vi "App - analyze RUS V6.vi"() -> ()   [LabVIEW 2018] (continued)
ember_2014\\091714\\45.19600K_500_2500_2.10000V_0.00000T_Sep17-2014__13-27-32_001_091714.bin", "mod time(min)"=58230327.53333333, "file format"=enum."binary", "power(V)"=2.1, "Magn Field(T) "=0.0}, {"temperature"=45.12, "temperature str"="45.12000", "file path"=path "D:/Data/Ultrasound/LSCO/LSCO22__130814c/5_Cooling_2nd_try/September_2014/091714/45.12000K_500_2500_2.10000V_0.00000T_Sep17-2014__13-28-51_001_091714.bin", "last mod"=timestamp(3493819731 s since 1904-01-01), "file name str"="D:\\Data\\Ultrasound\\LSCO\\LSCO22__130814c\\5_Cooling_2nd_try\\September_2014\\091714\\45.12000K_500_2500_2.10000V_0.00000T_Sep17-2014__13-28-51_001_091714.bin", "mod time(min)"=58230328.85, "file format"=enum."binary", "power(V)"=2.1, "Magn Field(T) "=0.0}, {"temperature"=45.046, "temperature str"="45.04600", "file path"=path "D:/Data/Ultrasound/LSCO/LSCO22__130814c/5_Cooling_2nd_try/September_2014/091714/45.04600K_500_2500_2.10000V_0.00000T_Sep17-2014__13-30-10_001_091714.bin", "last mod"=timestamp(3493819810 s since 1904-01-01), "file name str"="D:\\Data\\Ultrasound\\LSCO\\LSCO22__130814c\\5_Cooling_2nd_try\\September_2014\\091714\\45.04600K_500_2500_2.10000V_0.00000T_Sep17-2014__13-30-10_001_091714.bin", "mod time(min)"=58230330.166666664, "file format"=enum."binary", "power(V)"=2.1, "Magn Field(T) "=0.0}, {"temperature"=44.972, "temperature str"="44.97200", "file path"=path "D:/Data/Ultrasound/LSCO/LSCO22__130814c/5_Cooling_2nd_try/September_2014/091714/44.97200K_500_2500_2.10000V_0.00000T_Sep17-2014__13-31-30_001_091714.bin", "last mod"=timestamp(3493819890 s since 1904-01-01), "file name str"="D:\\Data\\Ultrasound\\LSCO\\LSCO22__130814c\\5_Cooling_2nd_try\\September_2014\\091714\\44.97200K_500_2500_2.10000V_0.00000T_Sep17-2014__13-31-30_001_091714.bin", "mod time(min)"=58230331.5, "file format"=enum."binary", "power(V)"=2.1, "Magn Field(T) "=0.0}, {"temperature"=44.9, "temperature str"="44.90000", "file path"=path "D:/Data/Ultrasound/LSCO/LSCO22__130814c/5_Cooling_2nd_try/September_2014/091714/44.90000K_500_2500_2.10000V_0.00000T_Sep17-2014__13-32-49_001_091714.bin", "last mod"=timestamp(3493819969 s since 1904-01-01), "file name str"="D:\\Data\\Ultrasound\\LSCO\\LSCO22__130814c\\5_Cooling_2nd_try\\September_2014\\091714\\44.90000K_500_2500_2.10000V_0.00000T_Sep17-2014__13-32-49_001_091714.bin", "mod time(min)"=58230332.81666667, "file format"=enum."binary", "power(V)"=2.1, "Magn Field(T) "=0.0}, {"temperature"=44.826, "temperature str"="44.82600", "file path"=path "D:/Data/Ultrasound/LSCO/LSCO22__130814c/5_Cooling_2nd_try/September_2014/091714/44.82600K_500_2500_2.10000V_0.00000T_Sep17-2014__13-34-09_001_091714.bin", "last mod"=timestamp(3493820049 s since 1904-01-01), "file name str"="D:\\Data\\Ultrasound\\LSCO\\LSCO22__130814c\\5_Cooling_2nd_try\\September_2014\\091714\\44.82600K_500_2500_2.10000V_0.00000T_Sep17-2014__13-34-09_001_091714.bin", "mod time(min)"=58230334.15, "file format"=enum."binary", "power(V)"=2.1, "Magn Field(T) "=0.0}, {"temperature"=44.75, "temperature str"="44.75000", "file path"=path "D:/Data/Ultrasound/LSCO/LSCO22__130814c/5_Cooling_2nd_try/September_2014/091714/44.75000K_500_2500_2.10000V_0.00000T_Sep17-2014__13-35-28_001_091714.bin", "last mod"=timestamp(3493820128 s since 1904-01-01), "file name str"="D:\\Data\\Ultrasound\\LSCO\\LSCO22__130814c\\5_Cooling_2nd_try\\September_2014\\091714\\44.75000K_500_2500_2.10000V_0.00000T_Sep17-2014__13-35-28_001_091714.bin", "mod time(min)"=58230335.46666667, "file format"=enum."binary", "power(V)"=2.1, "Magn Field(T) "=0.0}, {"temperature"=44.678, "temperature str"="44.67800", "file path"=path "D:/Data/Ultrasound/LSCO/LSCO22__130814c/5_Cooling_2nd_try/September_2014/091714/44.67800K_500_2500_2.10000V_0.00000T_Sep17-2014__13-36-47_001_091714.bin", "last mod"=timestamp(3493820207 s since 1904-01-01), "file name str"="D:\\Data\\Ultrasound\\LSCO\\LSCO22__130814c\\5_Cooling_2nd_try\\September_2014\\091714\\44.67800K_500_2500_2.10000V_0.00000T_Sep17-2014__13-36-47_001_091714.bin", "mod time(min)"=58230336.78333333, "file format"=enum."binary", "power(V)"=2.1, "Magn Field(T) "=0.0}, {"temperature"=44.607, "temperature str"="44.60700", "file path"=path "D:/Data/Ultrasound/LSCO/LSCO22__130814c/5_Cooling_2nd_try/September_2014/091714/44.60700K_500_2500_2.10000V_0.00000T_Sep17-2014__13-38-07_001_091714.bin", "last mod"=timestamp(3493820287 s since 1904-01-01), "file name str"="D:\\Data\\Ultrasound\\LSCO\\LSCO22__130814c\\5_Cooling_2nd_try\\September_2014\\091714\\44.60700K_500_2500_2.10000V_0.00000T_Sep17-2014__13-38-07_001_091714.bin", "mod time(min)"=58230338.11666667, "file format"=enum."binary", "power(V)"=2.1, "Magn Field(T) "=0.0}, {"temperature"=44.533, "temperature str"="44.53300", "file path"=path "D:/Data/Ultrasound/LSCO/LSCO22__130814c/5_Cooling_2nd_try/September_2014/091714/44.53300K_500_2500_2.10000V_0.00000T_Sep17-2014__13-39-26_001_091714.bin", "last mod"=timestamp(3493820366 s since 1904-01-01), "file name str"="D:\\Data\\Ultrasound\\LSCO\\LSCO22__130814c\\5_Cooling_2nd_try\\September_2014\\091714\\44.53300K_500_2500_2.10000V_0.00000T_Sep17-2014__13-39-26_001_091714.bin", "mod time(min)"=58230339.43333333, "file format"=enum."binary", "power(V)"=2.1, "Magn Field(T) "=0.0}, {"temperature"=44.459, "temperature str"="44.45900", "file path"=path "D:/Data/Ultrasound/LSCO/LSCO22__130814c/5_Cooling_2nd_try/September_2014/091714/44.45900K_500_2500_2.10000V_0.00000T_Sep17-2014__13-40-45_001_091714.bin", "last mod"=timestamp(3493820445 s since 1904-01-01), "file name str"="D:\\Data\\Ultrasound\\LSCO\\LSCO22__130814c\\5_Cooling_2nd_try\\September_2014\\091714\\44.45900K_500_2500_2.10000V_0.00000T_Sep17-2014__13-40-45_001_091714.bin", "mod time(min)"=58230340.75, "file format"=enum."binary", "power(V)"=2.1, "Magn Field(T) "=0.0}, {"temperature"=44.38, "temperature str"="44.38000", "file path"=path "D:/Data/Ultrasound/LSCO/LSCO22__130814c/5_Cooling_2nd_try/September_2014/091714/44.38000K_500_2500_2.10000V_0.00000T_Sep17-2014__13-42-05_001_091714.bin", "last mod"=timestamp(3493820525 s since 1904-01-01), "file name str"="D:\\Data\\Ultrasound\\LSCO\\LSCO22__130814c\\5_Cooling_2nd_try\\September_2014\\091714\\44.38000K_500_2500_2.10000V_0.00000T_Sep17-2014__13-42-05_001_091714.bin", "mod time(min)"=58230342.083333336, "file format"=enum."binary", "power(V)"=2.1, "Magn Field(T) "=0.0}, {"temperature"=44.313, "temperature str"="44.31300", "file path"=path "D:/Data/Ultrasound/LSCO/LSCO22__130814c/5_Cooling_2nd_try/September_2014/091714/44.31300K_500_2500_2.10000V_0.00000T_Sep17-2014__13-43-24_001_091714.bin", "last mod"=timestamp(3493820604 s since 1904-01-01), "file name str"="D:\\Data\\Ultrasound\\LSCO\\LSCO22__130814c\\5_Cooling_2nd_try\\September_2014\\091714\\44.31300K_500_2500_2.10000V_0.00000T_Sep17-2014__13-43-24_001_091714.bin", "mod time(min)"=58230343.4, "file format"=enum."binary", "power(V)"=2.1, "Magn Field(T) "=0.0}, {"temperature"=44.23, "temperature str"="44.23000", "file path"=path "D:/Data/Ultrasound/LSCO/LSCO22__130814c/5_Cooling_2nd_try/September_2014/091714/44.23000K_500_2500_2.10000V_0.00000T_Sep17-2014__13-44-44_001_091714.bin", "last mod"=timestamp(3493820684 s since 1904-01-01), "file name str"="D:\\Data\\Ultrasound\\LSCO\\LSCO22__130814c\\5_Cooling_2nd_try\\September_2014\\091714\\44.23000K_500_2500_2.10000V_0.00000T_Sep17-2014__13-44-44_001_091714.bin", "mod time(min)"=58230344.733333334, "file format"=enum."binary", "power(V)"=2.1, "Magn Field(T) "=0.0}, {"temperature"=44.154, "temperature str"="44.15400", "file path"=path "D:/Data/Ultrasound/LSCO/LSCO22__130814c/5_Cooling_2nd_try/September_2014/091714/44.15400K_500_2500_2.10000V_0.00000T_Sep17-2014__13-46-03_001_091714.bin", "last mod"=timestamp(3493820763 s since 1904-01-01), "file name str"="D:\\Data\\Ultrasound\\LSCO\\LSCO22__130814c\\5_Cooling_2nd_try\\September_2014\\091714\\44.15400K_500_2500_2.10000V_0.00000T_Sep17-2014__13-46-03_001_091714.bin", "mod time(min)"=58230346.05, "file format"=enum."binary", "power(V)"=2.1, "Magn Field(T) "=0.0}, {"temperature"=44.084, "temperature str"="44.08400", "file path"=path "D:/Data/Ultrasound/LSCO/LSCO22__130814c/5_Cooling_2nd_try/September_2014/091714/44.08400K_500_2500_2.10000V_0.00000T_Sep17-2014__13-47-22_001_091714.bin", "last mod"=timestamp(3493820842 s since 1904-01-01), "file name str"="D:\\Data\\Ultrasound\\LSCO\\LSCO22__130814c\\5_Cooling_2nd_try\\September_2014\\091714\\44.08400K_500_2500_2.10000V_0.00000T_Sep17-2014__13-47-22_001_091714.bin", "mod time(min)"=58230347.36666667, "file format"=enum."binary", "power(V)"=2.1, "Magn Field(T) "=0.0}, {"temperature"=44.009, "temperature str"="44.00900", "file path"=path "D:/Data/Ultrasound/LSCO/LSCO22__130814c/5_Cooling_2nd_try/September_2014/091714/44.00900K_500_2500_2.10000V_0.00000T_Sep17-2014__13-48-42_001_091714.bin", "last mod"=timestamp(3493820922 s since 1904-01-01), "file name str"="D:\\Data\\Ultrasound\\LSCO\\LSCO22__130814c\\5_Cooling_2nd_try\\September_2014\\091714\\44.00900K_500_2500_2.10000V_0.00000T_Sep17-2014__13-48-42_001_091714.bin", "mod time(min)"=58230348.7, "file format"=enum."binary", "power(V)"=2.1, "Magn Field(T) "=0.0}, {"temperature"=43.936, "temperature str"="43.93600", "file path"=path "D:/Data/Ultrasound/LSCO/LSCO22__130814c/5_Cooling_2nd_try/September_2014/091714/43.93600K_500_2500_2.10000V_0.00000T_Sep17-2014__13-50-01_001_091714.bin", "last mod"=timestamp(3493821001 s since 1904-01-01), "file name str"="D:\\Data\\Ultrasound\\LSCO\\LSCO22__130814c\\5_Cooling_2nd_try\\September_2014\\091714\\43.93600K_500_2500_2.10000V_0.00000T_Sep17-2014__13-50-01_001_091714.bin", "mod time(min)"=58230350.016666666, "file format"=enum."binary", "power(V)"=2.1, "Magn Field(T) "=0.0}, {"temperature"=43.859, "temperature str"="43.85900", "file path"=path "D:/Data/Ultrasound/LSCO/LSCO22__130814c/5_Cooling_2nd_try/September_2014/091714/43.85900K_500_2500_2.10000V_0.00000T_Sep17-2014__13-51-20_001_091714.bin", "last mod"=timestamp(3493821080 s since 1904-01-01), "file name str"="D:\\Data\\Ultrasound\\LSCO\\LSCO22__130814c\\5_Cooling_2nd_try\\September_2014\\091714\\43.85900K_500_2500_2.10000V_0.00000T_Sep17-2014__13-51-20_001_091714.bin", "mod time(min)"=58230351.333333336, "file format"=enum."binary", "power(V)"=2.1, "Magn Field(T) "=0.0}, {"temperature"=43.784, "temperature str"="43.78400", "file path"=path "D:/Data/Ultrasound/LSCO/LSCO22__130814c/5_Cooling_2nd_try/September_2014/091714/43.78400K_500_2500_2.10000V_0.00000T_Sep17-2014__13-52-40_001_091714.bin", "last mod"=timestamp(3493821160 s since 1904-01-01), "file name str"="D:\\Data\\Ultrasound\\LSCO\\LSCO22__130814c\\5_Cooling_2nd_try\\September_2014\\091714\\43.78400K_500_2500_2.10000V_0.00000T_Sep17-2014__13-52-40_001_091714.bin", "mod time(min)"=58230352.666666664, "file format"=enum."binary", "power(V)"=2.1, "Magn Field(T) "=0.0}, {"temperature"=43.711, "temperature str"="43.71100", "file path"=path "D:/Data/Ultrasound/LSCO/LSCO22__130814c/5_Cooling_2nd_try/September_2014/091714/43.71100K_500_2500_2.10000V_0.00000T_Sep17-2014__13-53-59_001_091714.bin", "last mod"=timestamp(3493821239 s since 1904-01-01), "file name str"="D:\\Data\\Ultrasound\\LSCO\\LSCO22__130814c\\5_Cooling_2nd_try\\September_2014\\091714\\43.71100K_500_2500_2.10000V_0.00000T_Sep17-2014__13-53-59_001_091714.bin", "mod time(min)"=58230353.983333334, "file format"=enum."binary", "power(V)"=2.1, "Magn Field(T) "=0.0}, {"temperature"=43.633, "temperature str"="43.63300", "file path"=path "D:/Data/Ultrasound/LSCO/LSCO22__130814c/5_Cooling_2nd_try/September_2014/091714/43.63300K_500_2500_2.10000V_0.00000T_Sep17-2014__13-55-19_001_091714.bin", "last mod"=timestamp(3493821319 s since 1904-01-01), "file name str"="D:\\Data\\Ultrasound\\LSCO\\LSCO22__130814c\\5_Cooling_2nd_try\\September_2014\\091714\\43.63300K_500_2500_2.10000V_0.00000T_Sep17-2014__13-55-19_001_091714.bin", "mod time(min)"=58230355.31666667, "file format"=enum."binary", "power(V)"=2.1, "Magn Field(T) "=0.0}, {"temperature"=43.561, "temperature str"="43.56100", "file path"=path "D:/Data/Ultrasound/LSCO/LSCO22__130814c/5_Cooling_2nd_try/September_2014/091714/43.56100K_500_2500_2.10000V_0.00000T_Sep17-2014__13-56-38_001_091714.bin", "last mod"=timestamp(3493821398 s since 1904-01-01), "file name str"="D:\\Data\\Ultrasound\\LSCO\\LSCO22__130814c\\5_Cooling_2nd_try\\September_2014\\091714\\43.56100K_500_2500_2.10000V_0.00000T_Sep17-2014__13-56-38_001_091714.bin", "mod time(min)"=58230356.63333333, "file format"=enum."binary", "power(V)"=2.1, "Magn Field(T) "=0.0}, {"temperature"=43.487, "temperature str"="43.48700", "file path"=path "D:/Data/Ultrasound/LSCO/LSCO22__130814c/5_Cooling_2nd_try/September_2014/091714/43.48700K_500_2500_2.10000V_0.00000T_Sep17-2014__13-57-57_001_091714.bin", "last mod"=timestamp(3493821477 s since 1904-01-01), "file name str"="D:\\Data\\Ultrasound\\LSCO\\LSCO22__130814c\\5_Cooling_2nd_try\\September_2014\\091714\\43.48700K_500_2500_2.10000V_0.00000T_Sep17-2014__13-57-57_001_091714.bin", "mod time(min)"=58230357.95, "file format"=enum."binary", "power(V)"=2.1, "Magn Field(T) "=0.0}, {"temperature"=43.408, "temperature str"="43.40800", "file path"=path "D:/Data/Ultrasound/LSCO/LSCO22__130814c/5_Cooling_2nd_try/September_2014/091714/43.40800K_500_2500_2.10000V_0.00000T_Sep17-2014__13-59-17_001_091714.bin", "last mod"=timestamp(3493821557 s since 1904-01-01), "file name str"="D:\\Data\\Ultrasound\\LSCO\\LSCO22__130814c\\5_Cooling_2nd_try\\September_2014\\091714\\43.40800K_500_2500_2.10000V_0.00000T_Sep17-2014__13-59-17_001_091714.bin", "mod time(min)"=58230359.28333333, "file format"=enum."binary", "power(V)"=2.1, "Magn Field(T) "=0.0}, {"temperature"=43.333, "temperature str"="43.33300", "file path"=path "D:/Data/Ultrasound/LSCO/LSCO22__130814c/5_Cooling_2nd_try/September_2014/091714/43.33300K_500_2500_2.10000V_0.00000T_Sep17-2014__14-00-36_001_091714.bin", "last mod"=timestamp(3493821636 s since 1904-01-01), "file name str"="D:\\Data\\Ultrasound\\LSCO\\LSCO22__130814c\\5_Cooling_2nd_try\\September_2014\\091714\\43.33300K_500_2500_2.10000V_0.00000T_Sep17-2014__14-00-36_001_091714.bin", "mod time(min)"=58230360.6, "file format"=enum."binary", "power(V)"=2.1, "Magn Field(T) "=0.0}, {"temperature"=43.259, "temperature str"="43.25900", "file path"=path "D:/Data/Ultrasound/LSCO/LSCO22__130814c/5_Cooling_2nd_try/September_2014/091714/43.25900K_500_2500_2.10000V_0.00000T_Sep17-2014__14-01-55_001_091714.bin", "last mod"=timestamp(3493821715 s since 1904-01-01), "file name str"="D:\\Data\\Ultrasound\\LSCO\\LSCO22__130814c\\5_Cooling_2nd_try\\September_2014\\091714\\43.25900K_500_2500_2.10000V_0.00000T_Sep17-2014__14-01-55_001_091714.bin", "mod time(min)"=58230361.916666664, "file format"=enum."binary", "power(V)"=2.1, "Magn Field(T) "=0.0}, {"temperature"=43.185, "temperature str"="43.18500", "file path"=path "D:/Data/Ultrasound/LSCO/LSCO22__130814c/5_Cooling_2nd_try/September_2014/091714/43.18500K_500_2500_2.10000V_0.00000T_Sep17-2014__14-03-15_001_091714.bin", "last mod"=timestamp(3493821795 s since 1904-01-01), "file name str"="D:\\Data\\Ultrasound\\LSCO\\LSCO22__130814c\\5_Cooling_2nd_try\\September_2014\\091714\\43.18500K_500_2500_2.10000V_0.00000T_Sep17-2014__14-03-15_001_091714.bin", "mod time(min)"=58230363.25, "file format"=enum."binary", "power(V)"=2.1, "Magn Field(T) "=0.0}, {"temperature"=43.113, "temperature str"="43.11300", "file path"=path "D:/Data/Ultrasound/LSCO/LSCO22__130814c/5_Cooling_2nd_try/September_2014/091714/43.11300K_500_2500_2.10000V_0.00000T_Sep17-2014__14-04-34_001_091714.bin", "last mod"=timestamp(3493821874 s since 1904-01-01), "file name str"="D:\\Data\\Ultrasound\\LSCO\\LSCO22__130814c\\5_Cooling_2nd_try\\September_2014\\091714\\43.11300K_500_2500_2.10000V_0.00000T_Sep17-2014__14-04-34_001_091714.bin", "mod time(min)"=58230364.56666667, "file format"=enum."binary", "power(V)"=2.1, "Magn Field(T) "=0.0}, {"temperature"=43.031, "temperature str"="43.03100", "file path"=path "D:/Data/Ultrasound/LSCO/LSCO22__130814c/5_Cooling_2nd_try/September_2014/091714/43.03100K_500_2500_2.10000V_0.00000T_Sep17-2014__14-05-54_001_091714.bin", "last mod"=timestamp(3493821954 s since 1904-01-01), "file name str"="D:\\Data\\Ultrasound\\LSCO\\LSCO22__130814c\\5_Cooling_2nd_try\\September_2014\\091714\\43.03100K_500_2500_2.10000V_0.00000T_Sep17-2014__14-05-54_001_091714.bin", "mod time(min)"=58230365.9, "file format"=enum."binary", "power(V)"=2.1, "Magn Field(T) "=0.0}, {"temperature"=42.958, "temperature str"="42.95800", "file path"=path "D:/Data/Ultrasound/LSCO/LSCO22__130814c/5_Cooling_2nd_try/September_2014/091714/42.95800K_500_2500_2.10000V_0.00000T_Sep17-2014__14-07-13_001_091714.bin", "last mod"=timestamp(3493822033 s since 1904-01-01), "file name str"="D:\\Data\\Ultrasound\\LSCO\\LSCO22__130814c\\5_Cooling_2nd_try\\September_2014\\091714\\42.95800K_500_2500_2.10000V_0.00000T_Sep17-2014__14-07-13_001_091714.bin", "mod time(min)"=58230367.21666667, "file format"=enum."binary", "power(V)"=2.1, "Magn Field(T) "=0.0}, {"temperature"=42.88, "temperature str"="42.88000", "file path"=path "D:/Data/Ultrasound/LSCO/LSCO22__130814c/5_Cooling_2nd_try/September_2014/091714/42.88000K_500_2500_2.10000V_0.00000T_Sep17-2014__14-08-32_001_091714.bin", "last mod"=timestamp(3493822112 s since 1904-01-01), "file name str"="D:\\Data\\Ultrasound\\LSCO\\LSCO22__130814c\\5_Cooling_2nd_try\\September_2014\\091714\\42.88000K_500_2500_2.10000V_0.00000T_Sep17-2014__14-08-32_001_091714.bin", "mod time(min)"=58230368.53333333, "file format"=enum."binary", "power(V)"=2.1, "Magn Field(T) "=0.0}, {"temperature"=42.806, "temperature str"="42.80600", "file path"=path "D:/Data/Ultrasound/LSCO/LSCO22__130814c/5_Cooling_2nd_try/September_2014/091714/42.80600K_500_2500_2.10000V_0.00000T_Sep17-2014__14-09-52_001_091714.bin", "last mod"=timestamp(3493822192 s since 1904-01-01), "file name str"="D:\\Data\\Ultrasound\\LSCO\\LSCO22__130814c\\5_Cooling_2nd_try\\September_2014\\091714\\42.80600K_500_2500_2.10000V_0.00000T_Sep17-2014__14-09-52_001_091714.bin", "mod time(min)"=58230369.86666667, "file format"=enum."binary", "power(V)"=2.1, "Magn Field(T) "=0.0}, {"temperature"=42.73, "temperature str"="42.73000", "file path"=path "D:/Data/Ultrasound/LSCO/LSCO22__130814c/5_Cooling_2nd_try/September_2014/091714/42.73000K_500_2500_2.10000V_0.00000T_Sep17-2014__14-11-11_001_091714.bin", "last mod"=timestamp(3493822271 s since 1904-01-01), "file name str"="D:\\Data\\Ultrasound\\LSCO\\LSCO22__130814c\\5_Cooling_2nd_try\\September_2014\\091714\\42.73000K_500_2500_2.10000V_0.00000T_Sep17-2014__14-11-11_001_091714.bin", "mod time(min)"=58230371.18333333, "file format"=enum."binary", "power(V)"=2.1, "Magn Field(T) "=0.0}, {"temperature"=42.653, "temperature str"="42.65300", "file path"=path "D:/Data/Ultrasound/LSCO/LSCO22__130814c/5_Cooling_2nd_try/September_2014/091714/42.65300K_500_2500_2.10000V_0.00000T_Sep17-2014__14-12-30_001_091714.bin", "last mod"=timestamp(3493822350 s since 1904-01-01), "file name str"="D:\\Data\\Ultrasound\\LSCO\\LSCO22__130814c\\5_Cooling_2nd_try\\September_2014\\091714\\42.65300K_500_2500_2.10000V_0.00000T_Sep17-2014__14-12-30_001_091714.bin", "mod time(min)"=58230372.5, "file format"=enum."binary", "power(V)"=2.1, "Magn Field(T) "=0.0}, {"temperature"=42.575, "temperature str"="42.57500", "file path"=path "D:/Data/Ultrasound/LSCO/LSCO22__130814c/5_Cooling_2nd_try/September_2014/091714/42.57500K_500_2500_2.10000V_0.00000T_Sep17-2014__14-13-50_001_091714.bin", "last mod"=timestamp(3493822430 s since 1904-01-01), "file name str"="D:\\Data\\Ultrasound\\LSCO\\LSCO22__130814c\\5_Cooling_2nd_try\\September_2014\\091714\\42.57500K_500_2500_2.10000V_0.00000T_Sep17-2014__14-13-50_001_091714.bin", "mod time(min)"=58230373.833333336, "file format"=enum."binary", "power(V)"=2.1, "Magn Field(T) "=0.0}, {"temperature"=42.498, "temperature str"="42.49800", "file path"=path "D:/Data/Ultrasound/LSCO/LSCO22__130814c/5_Cooling_2nd_try/September_2014/091714/42.49800K_500_2500_2.10000V_0.00000T_Sep17-2014__14-15-09_001_091714.bin", "last mod"=timestamp(3493822509 s since 1904-01-01), "file name str"="D:\\Data\\Ultrasound\\LSCO\\LSCO22__130814c\\5_Cooling_2nd_try\\September_2014\\091714\\42.49800K_500_2500_2.10000V_0.00000T_Sep17-2014__14-15-09_001_091714.bin", "mod time(min)"=58230375.15, "file format"=enum."binary", "power(V)"=2.1, "Magn Field(T) "=0.0}, {"temperature"=42.427, "temperature str"="42.42700", "file path"=path "D:/Data/Ultrasound/LSCO/LSCO22__130814c/5_Cooling_2nd_try/September_2014/091714/42.42700K_500_2500_2.10000V_0.00000T_Sep17-2014__14-16-29_001_091714.bin", "last mod"=timestamp(3493822589 s since 1904-01-01), "file name str"="D:\\Data\\Ultrasound\\LSCO\\LSCO22__130814c\\5_Cooling_2nd_try\\September_2014\\091714\\42.42700K_500_2500_2.10000V_0.00000T_Sep17-2014__14-16-29_001_091714.bin", "mod time(min)"=58230376.483333334, "file format"=enum."binary", "power(V)"=2.1, "Magn Field(T) "=0.0}, {"temperature"=42.347, "temperature str"="42.34700", "file path"=path "D:/Data/Ultrasound/LSCO/LSCO22__130814c/5_Cooling_2nd_try/September_2014/091714/42.34700K_500_2500_2.10000V_0.00000T_Sep17-2014__14-17-48_001_091714.bin", "last mod"=timestamp(3493822668 s since 1904-01-01), "file name str"="D:\\Data\\Ultrasound\\LSCO\\LSCO22__130814c\\5_Cooling_2nd_try\\September_2014\\091714\\42.34700K_500_2500_2.10000V_0.00000T_Sep17-2014__14-17-48_001_091714.bin", "mod time(min)"=58230377.8, "file format"=enum."binary", "power(V)"=2.1, "Magn Field(T) "=0.0}, {"temperature"=42.268, "temperature str"="42.26800", "file path"=path "D:/Data/Ultrasound/LSCO/LSCO22__130814c/5_Cooling_2nd_try/September_2014/091714/42.26800K_500_2500_2.10000V_0.00000T_Sep17-2014__14-19-07_001_091714.bin", "last mod"=timestamp(3493822747 s since 1904-01-01), "file name str"="D:\\Data\\Ultrasound\\LSCO\\LSCO22__130814c\\5_Cooling_2nd_try\\September_2014\\091714\\42.26800K_500_2500_2.10000V_0.00000T_Sep17-2014__14-19-07_001_091714.bin", "mod time(min)"=58230379.11666667, "file format"=enum."binary", "power(V)"=2.1, "Magn Field(T) "=0.0}, {"temperature"=42.196, "temperature str"="42.19600", "file path"=path "D:/Data/Ultrasound/LSCO/LSCO22__130814c/5_Cooling_2nd_try/September_2014/091714/42.19600K_500_2500_2.10000V_0.00000T_Sep17-2014__14-20-27_001_091714.bin", "last mod"=timestamp(3493822827 s since 1904-01-01), "file name str"="D:\\Data\\Ultrasound\\LSCO\\LSCO22__130814c\\5_Cooling_2nd_try\\September_2014\\091714\\42.19600K_500_2500_2.10000V_0.00000T_Sep17-2014__14-20-27_001_091714.bin", "mod time(min)"=58230380.45, "file format"=enum."binary", "power(V)"=2.1, "Magn Field(T) "=0.0}, {"temperature"=42.117, "temperature str"="42.11700", "file path"=path "D:/Data/Ultrasound/LSCO/LSCO22__130814c/5_Cooling_2nd_try/September_2014/091714/42.11700K_500_2500_2.10000V_0.00000T_Sep17-2014__14-21-46_001_091714.bin", "last mod"=timestamp(3493822906 s since 1904-01-01), "file name str"="D:\\Data\\Ultrasound\\LSCO\\LSCO22__130814c\\5_Cooling_2nd_try\\September_2014\\091714\\42.11700K_500_2500_2.10000V_0.00000T_Sep17-2014__14-21-46_001_091714.bin", "mod time(min)"=58230381.766666666, "file format"=enum."binary", "power(V)"=2.1, "Magn Field(T) "=0.0}, {"temperature"=42.038, "temperature str"="42.03800", "file path"=path "D:/Data/Ultrasound/LSCO/LSCO22__130814c/5_Cooling_2nd_try/September_2014/091714/42.03800K_500_2500_2.10000V_0.00000T_Sep17-2014__14-23-05_001_091714.bin", "last mod"=timestamp(3493822985 s since 1904-01-01), "file name str"="D:\\Data\\Ultrasound\\LSCO\\LSCO22__130814c\\5_Cooling_2nd_try\\September_2014\\091714\\42.03800K_500_2500_2.10000V_0.00000T_Sep17-2014__14-23-05_001_091714.bin", "mod time(min)"=58230383.083333336, "file format"=enum."binary", "power(V)"=2.1, "Magn Field(T) "=0.0}, {"temperature"=41.963, "temperature str"="41.96300", "file path"=path "D:/Data/Ultrasound/LSCO/LSCO22__130814c/5_Cooling_2nd_try/September_2014/091714/41.96300K_500_2500_2.10000V_0.00000T_Sep17-2014__14-24-25_001_091714.bin", "last mod"=timestamp(3493823065 s since 1904-01-01), "file name str"="D:\\Data\\Ultrasound\\LSCO\\LSCO22__130814c\\5_Cooling_2nd_try\\September_2014\\091714\\41.96300K_500_2500_2.10000V_0.00000T_Sep17-2014__14-24-25_001_091714.bin", "mod time(min)"=58230384.416666664, "file format"=enum."binary", "power(V)"=2.1, "Magn Field(T) "=0.0}, {"temperature"=41.884, "temperature str"="41.88400", "file path"=path "D:/Data/Ultrasound/LSCO/LSCO22__130814c/5_Cooling_2nd_try/September_2014/091714/41.88400K_500_2500_2.10000V_0.00000T_Sep17-2014__14-25-44_001_091714.bin", "last mod"=timestamp(3493823144 s since 1904-01-01), "file name str"="D:\\Data\\Ultrasound\\LSCO\\LSCO22__130814c\\5_Cooling_2nd_try\\September_2014\\091714\\41.88400K_500_2500_2.10000V_0.00000T_Sep17-2014__14-25-44_001_091714.bin", "mod time(min)"=58230385.733333334, "file format"=enum."binary", "power(V)"=2.1, "Magn Field(T) "=0.0}, {"temperature"=41.812, "temperature str"="41.81200", "file path"=path "D:/Data/Ultrasound/LSCO/LSCO22__130814c/5_Cooling_2nd_try/September_2014/091714/41.81200K_500_2500_2.10000V_0.00000T_Sep17-2014__14-27-12_001_091714.bin", "last mod"=timestamp(3493823232 s since 1904-01-01), "file name str"="D:\\Data\\Ultrasound\\LSCO\\LSCO22__130814c\\5_Cooling_2nd_try\\September_2014\\091714\\41.81200K_500_2500_2.10000V_0.00000T_Sep17-2014__14-27-12_001_091714.bin", "mod time(min)"=58230387.2, "file format"=enum."binary", "power(V)"=2.1, "Magn Field(T) "=0.0}, {"temperature"=41.716, "temperature str"="41.71600", "file path"=path "D:/Data/Ultrasound/LSCO/LSCO22__130814c/5_Cooling_2nd_try/September_2014/091714/41.71600K_500_2500_2.10000V_0.00000T_Sep17-2014__14-28-31_001_091714.bin", "last mod"=timestamp(3493823311 s since 1904-01-01), "file name str"="D:\\Data\\Ultrasound\\LSCO\\LSCO22__130814c\\5_Cooling_2nd_try\\September_2014\\091714\\41.71600K_500_2500_2.10000V_0.00000T_Sep17-2014__14-28-31_001_091714.bin", "mod time(min)"=58230388.516666666, "file format"=enum."binary", "power(V)"=2.1, "Magn Field(T) "=0.0}, {"temperature"=41.641, "temperature str"="41.64100", "file path"=path "D:/Data/Ultrasound/LSCO/LSCO22__130814c/5_Cooling_2nd_try/September_2014/091714/41.64100K_500_2500_2.10000V_0.00000T_Sep17-2014__14-29-50_001_091714.bin", "last mod"=timestamp(3493823390 s since 1904-01-01), "file name str"="D:\\Data\\Ultrasound\\LSCO\\LSCO22__130814c\\5_Cooling_2nd_try\\September_2014\\091714\\41.64100K_500_2500_2.10000V_0.00000T_Sep17-2014__14-29-50_001_091714.bin", "mod time(min)"=58230389.833333336, "file format"=enum."binary", "power(V)"=2.1, "Magn Field(T) "=0.0}, {"temperature"=41.564, "temperature str"="41.56400", "file path"=path "D:/Data/Ultrasound/LSCO/LSCO22__130814c/5_Cooling_2nd_try/September_2014/091714/41.56400K_500_2500_2.10000V_0.00000T_Sep17-2014__14-31-10_001_091714.bin", "last mod"=timestamp(3493823470 s since 1904-01-01), "file name str"="D:\\Data\\Ultrasound\\LSCO\\LSCO22__130814c\\5_Cooling_2nd_try\\September_2014\\091714\\41.56400K_500_2500_2.10000V_0.00000T_Sep17-2014__14-31-10_001_091714.bin", "mod time(min)"=58230391.166666664, "file format"=enum."binary", "power(V)"=2.1, "Magn Field(T) "=0.0}, {"temperature"=41.488, "temperature str"="41.48800", "file path"=path "D:/Data/Ultrasound/LSCO/LSCO22__130814c/5_Cooling_2nd_try/September_2014/091714/41.48800K_500_2500_2.10000V_0.00000T_Sep17-2014__14-32-29_001_091714.bin", "last mod"=timestamp(3493823549 s since 1904-01-01), "file name str"="D:\\Data\\Ultrasound\\LSCO\\LSCO22__130814c\\5_Cooling_2nd_try\\September_2014\\091714\\41.48800K_500_2500_2.10000V_0.00000T_Sep17-2014__14-32-29_001_091714.bin", "mod time(min)"=58230392.483333334, "file format"=enum."binary", "power(V)"=2.1, "Magn Field(T) "=0.0}, {"temperature"=41.411, "temperature str"="41.41100", "file path"=path "D:/Data/Ultrasound/LSCO/LSCO22__130814c/5_Cooling_2nd_try/September_2014/091714/41.41100K_500_2500_2.10000V_0.00000T_Sep17-2014__14-33-49_001_091714.bin", "last mod"=timestamp(3493823629 s since 1904-01-01), "file name str"="D:\\Data\\Ultrasound\\LSCO\\LSCO22__130814c\\5_Cooling_2nd_try\\September_2014\\091714\\41.41100K_500_2500_2.10000V_0.00000T_Sep17-2014__14-33-49_001_091714.bin", "mod time(min)"=58230393.81666667, "file format"=enum."binary", "power(V)"=2.1, "Magn Field(T) "=0.0}, {"temperature"=41.326, "temperature str"="41.32600", "file path"=path "D:/Data/Ultrasound/LSCO/LSCO22__130814c/5_Cooling_2nd_try/September_2014/091714/41.32600K_500_2500_2.10000V_0.00000T_Sep17-2014__14-35-08_001_091714.bin", "last mod"=timestamp(3493823708 s since 1904-01-01), "file name str"="D:\\Data\\Ultrasound\\LSCO\\LSCO22__130814c\\5_Cooling_2nd_try\\September_2014\\091714\\41.32600K_500_2500_2.10000V_0.00000T_Sep17-2014__14-35-08_001_091714.bin", "mod time(min)"=58230395.13333333, "file format"=enum."binary", "power(V)"=2.1, "Magn Field(T) "=0.0}, {"temperature"=41.255, "temperature str"="41.25500", "file path"=path "D:/Data/Ultrasound/LSCO/LSCO22__130814c/5_Cooling_2nd_try/September_2014/091714/41.25500K_500_2500_2.10000V_0.00000T_Sep17-2014__14-36-27_001_091714.bin", "last mod"=timestamp(3493823787 s since 1904-01-01), "file name str"="D:\\Data\\Ultrasound\\LSCO\\LSCO22__130814c\\5_Cooling_2nd_try\\September_2014\\091714\\41.25500K_500_2500_2.10000V_0.00000T_Sep17-2014__14-36-27_001_091714.bin", "mod time(min)"=58230396.45, "file format"=enum."binary", "power(V)"=2.1, "Magn Field(T) "=0.0}, {"temperature"=41.174, "temperature str"="41.17400", "file path"=path "D:/Data/Ultrasound/LSCO/LSCO22__130814c/5_Cooling_2nd_try/September_2014/091714/41.17400K_500_2500_2.10000V_0.00000T_Sep17-2014__14-37-47_001_091714.bin", "last mod"=timestamp(3493823867 s since 1904-01-01), "file name str"="D:\\Data\\Ultrasound\\LSCO\\LSCO22__130814c\\5_Cooling_2nd_try\\September_2014\\091714\\41.17400K_500_2500_2.10000V_0.00000T_Sep17-2014__14-37-47_001_091714.bin", "mod time(min)"=58230397.78333333, "file format"=enum."binary", "power(V)"=2.1, "Magn Field(T) "=0.0}, {"temperature"=41.098, "temperature str"="41.09800", "file path"=path "D:/Data/Ultrasound/LSCO/LSCO22__130814c/5_Cooling_2nd_try/September_2014/091714/41.09800K_500_2500_2.10000V_0.00000T_Sep17-2014__14-39-06_001_091714.bin", "last mod"=timestamp(3493823946 s since 1904-01-01), "file name str"="D:\\Data\\Ultrasound\\LSCO\\LSCO22__130814c\\5_Cooling_2nd_try\\September_2014\\091714\\41.09800K_500_2500_2.10000V_0.00000T_Sep17-2014__14-39-06_001_091714.bin", "mod time(min)"=58230399.1, "file format"=enum."binary", "power(V)"=2.1, "Magn Field(T) "=0.0}, {"temperature"=41.017, "temperature str"="41.01700", "file path"=path "D:/Data/Ultrasound/LSCO/LSCO22__130814c/5_Cooling_2nd_try/September_2014/091714/41.01700K_500_2500_2.10000V_0.00000T_Sep17-2014__14-40-25_001_091714.bin", "last mod"=timestamp(3493824025 s since 1904-01-01), "file name str"="D:\\Data\\Ultrasound\\LSCO\\LSCO22__130814c\\5_Cooling_2nd_try\\September_2014\\091714\\41.01700K_500_2500_2.10000V_0.00000T_Sep17-2014__14-40-25_001_091714.bin", "mod time(min)"=58230400.416666664, "file format"=enum."binary", "power(V)"=2.1, "Magn Field(T) "=0.0}, {"temperature"=40.94, "temperature str"="40.94000", "file path"=path "D:/Data/Ultrasound/LSCO/LSCO22__130814c/5_Cooling_2nd_try/September_2014/091714/40.94000K_500_2500_2.10000V_0.00000T_Sep17-2014__14-41-45_001_091714.bin", "last mod"=timestamp(3493824105 s since 1904-01-01), "file name str"="D:\\Data\\Ultrasound\\LSCO\\LSCO22__130814c\\5_Cooling_2nd_try\\September_2014\\091714\\40.94000K_500_2500_2.10000V_0.00000T_Sep17-2014__14-41-45_001_091714.bin", "mod time(min)"=58230401.75, "file format"=enum."binary", "power(V)"=2.1, "Magn Field(T) "=0.0}, {"temperature"=40.861, "temperature str"="40.86100", "file path"=path "D:/Data/Ultrasound/LSCO/LSCO22__130814c/5_Cooling_2nd_try/September_2014/091714/40.86100K_500_2500_2.10000V_0.00000T_Sep17-2014__14-43-04_001_091714.bin", "last mod"=timestamp(3493824184 s since 1904-01-01), "file name str"="D:\\Data\\Ultrasound\\LSCO\\LSCO22__130814c\\5_Cooling_2nd_try\\September_2014\\091714\\40.86100K_500_2500_2.10000V_0.00000T_Sep17-2014__14-43-04_001_091714.bin", "mod time(min)"=58230403.06666667, "file format"=enum."binary", "power(V)"=2.1, "Magn Field(T) "=0.0}, {"temperature"=40.779, "temperature str"="40.77900", "file path"=path "D:/Data/Ultrasound/LSCO/LSCO22__130814c/5_Cooling_2nd_try/September_2014/091714/40.77900K_500_2500_2.10000V_0.00000T_Sep17-2014__14-44-24_001_091714.bin", "last mod"=timestamp(3493824264 s since 1904-01-01), "file name str"="D:\\Data\\Ultrasound\\LSCO\\LSCO22__130814c\\5_Cooling_2nd_try\\September_2014\\091714\\40.77900K_500_2500_2.10000V_0.00000T_Sep17-2014__14-44-24_001_091714.bin", "mod time(min)"=58230404.4, "file format"=enum."binary", "power(V)"=2.1, "Magn Field(T) "=0.0}, {"temperature"=40.702, "temperature str"="40.70200", "file path"=path "D:/Data/Ultrasound/LSCO/LSCO22__130814c/5_Cooling_2nd_try/September_2014/091714/40.70200K_500_2500_2.10000V_0.00000T_Sep17-2014__14-45-43_001_091714.bin", "last mod"=timestamp(3493824343 s since 1904-01-01), "file name str"="D:\\Data\\Ultrasound\\LSCO\\LSCO22__130814c\\5_Cooling_2nd_try\\September_2014\\091714\\40.70200K_500_2500_2.10000V_0.00000T_Sep17-2014__14-45-43_001_091714.bin", "mod time(min)"=58230405.71666667, "file format"=enum."binary", "power(V)"=2.1, "Magn Field(T) "=0.0}, {"temperature"=40.621, "temperature str"="40.62100", "file path"=path "D:/Data/Ultrasound/LSCO/LSCO22__130814c/5_Cooling_2nd_try/September_2014/091714/40.62100K_500_2500_2.10000V_0.00000T_Sep17-2014__14-47-03_001_091714.bin", "last mod"=timestamp(3493824423 s since 1904-01-01), "file name str"="D:\\Data\\Ultrasound\\LSCO\\LSCO22__130814c\\5_Cooling_2nd_try\\September_2014\\091714\\40.62100K_500_2500_2.10000V_0.00000T_Sep17-2014__14-47-03_001_091714.bin", "mod time(min)"=58230407.05, "file format"=enum."binary", "power(V)"=2.1, "Magn Field(T) "=0.0}, {"temperature"=40.542, "temperature str"="40.54200", "file path"=path "D:/Data/Ultrasound/LSCO/LSCO22__130814c/5_Cooling_2nd_try/September_2014/091714/40.54200K_500_2500_2.10000V_0.00000T_Sep17-2014__14-48-22_001_091714.bin", "last mod"=timestamp(3493824502 s since 1904-01-01), "file name str"="D:\\Data\\Ultrasound\\LSCO\\LSCO22__130814c\\5_Cooling_2nd_try\\September_2014\\091714\\40.54200K_500_2500_2.10000V_0.00000T_Sep17-2014__14-48-22_001_091714.bin", "mod time(min)"=58230408.36666667, "file format"=enum."binary", "power(V)"=2.1, "Magn Field(T) "=0.0}, {"temperature"=40.463, "temperature str"="40.46300", "file path"=path "D:/Data/Ultrasound/LSCO/LSCO22__130814c/5_Cooling_2nd_try/September_2014/091714/40.46300K_500_2500_2.10000V_0.00000T_Sep17-2014__14-49-42_001_091714.bin", "last mod"=timestamp(3493824582 s since 1904-01-01), "file name str"="D:\\Data\\Ultrasound\\LSCO\\LSCO22__130814c\\5_Cooling_2nd_try\\September_2014\\091714\\40.46300K_500_2500_2.10000V_0.00000T_Sep17-2014__14-49-42_001_091714.bin", "mod time(min)"=58230409.7, "file format"=enum."binary", "power(V)"=2.1, "Magn Field(T) "=0.0}, {"temperature"=40.383, "temperature str"="40.38300", "file path"=path "D:/Data/Ultrasound/LSCO/LSCO22__130814c/5_Cooling_2nd_try/September_2014/091714/40.38300K_500_2500_2.10000V_0.00000T_Sep17-2014__14-51-01_001_091714.bin", "last mod"=timestamp(3493824661 s since 1904-01-01), "file name str"="D:\\Data\\Ultrasound\\LSCO\\LSCO22__130814c\\5_Cooling_2nd_try\\September_2014\\091714\\40.38300K_500_2500_2.10000V_0.00000T_Sep17-2014__14-51-01_001_091714.bin", "mod time(min)"=58230411.016666666, "file format"=enum."binary", "power(V)"=2.1, "Magn Field(T) "=0.0}, {"temperature"=40.311, "temperature str"="40.31100", "file path"=path "D:/Data/Ultrasound/LSCO/LSCO22__130814c/5_Cooling_2nd_try/September_2014/091714/40.31100K_500_2500_2.10000V_0.00000T_Sep17-2014__14-52-21_001_091714.bin", "last mod"=timestamp(3493824741 s since 1904-01-01), "file name str"="D:\\Data\\Ultrasound\\LSCO\\LSCO22__130814c\\5_Cooling_2nd_try\\September_2014\\091714\\40.31100K_500_2500_2.10000V_0.00000T_Sep17-2014__14-52-21_001_091714.bin", "mod time(min)"=58230412.35, "file format"=enum."binary", "power(V)"=2.1, "Magn Field(T) "=0.0}, {"temperature"=40.223, "temperature str"="40.22300", "file path"=path "D:/Data/Ultrasound/LSCO/LSCO22__130814c/5_Cooling_2nd_try/September_2014/091714/40.22300K_500_2500_2.10000V_0.00000T_Sep17-2014__14-53-40_001_091714.bin", "last mod"=timestamp(3493824820 s since 1904-01-01), "file name str"="D:\\Data\\Ultrasound\\LSCO\\LSCO22__130814c\\5_Cooling_2nd_try\\September_2014\\091714\\40.22300K_500_2500_2.10000V_0.00000T_Sep17-2014__14-53-40_001_091714.bin", "mod time(min)"=58230413.666666664, "file format"=enum."binary", "power(V)"=2.1, "Magn Field(T) "=0.0}, {"temperature"=40.145, "temperature str"="40.14500", "file path"=path "D:/Data/Ultrasound/LSCO/LSCO22__130814c/5_Cooling_2nd_try/September_2014/091714/40.14500K_500_2500_2.10000V_0.00000T_Sep17-2014__14-54-59_001_091714.bin", "last mod"=timestamp(3493824899 s since 1904-01-01), "file name str"="D:\\Data\\Ultrasound\\LSCO\\LSCO22__130814c\\5_Cooling_2nd_try\\September_2014\\091714\\40.14500K_500_2500_2.10000V_0.00000T_Sep17-2014__14-54-59_001_091714.bin", "mod time(min)"=58230414.983333334, "file format"=enum."binary", "power(V)"=2.1, "Magn Field(T) "=0.0}, {"temperature"=40.07, "temperature str"="40.07000", "file path"=path "D:/Data/Ultrasound/LSCO/LSCO22__130814c/5_Cooling_2nd_try/September_2014/091714/40.07000K_500_2500_2.10000V_0.00000T_Sep17-2014__14-56-19_001_091714.bin", "last mod"=timestamp(3493824979 s since 1904-01-01), "file name str"="D:\\Data\\Ultrasound\\LSCO\\LSCO22__130814c\\5_Cooling_2nd_try\\September_2014\\091714\\40.07000K_500_2500_2.10000V_0.00000T_Sep17-2014__14-56-19_001_091714.bin", "mod time(min)"=58230416.31666667, "file format"=enum."binary", "power(V)"=2.1, "Magn Field(T) "=0.0}, {"temperature"=39.984, "temperature str"="39.98400", "file path"=path "D:/Data/Ultrasound/LSCO/LSCO22__130814c/5_Cooling_2nd_try/September_2014/091714/39.98400K_500_2500_2.10000V_0.00000T_Sep17-2014__14-57-38_001_091714.bin", "last mod"=timestamp(3493825058 s since 1904-01-01), "file name str"="D:\\Data\\Ultrasound\\LSCO\\LSCO22__130814c\\5_Cooling_2nd_try\\September_2014\\091714\\39.98400K_500_2500_2.10000V_0.00000T_Sep17-2014__14-57-38_001_091714.bin", "mod time(min)"=58230417.63333333, "file format"=enum."binary", "power(V)"=2.1, "Magn Field(T) "=0.0}, {"temperature"=39.905, "temperature str"="39.90500", "file path"=path "D:/Data/Ultrasound/LSCO/LSCO22__130814c/5_Cooling_2nd_try/September_2014/091714/39.90500K_500_2500_2.10000V_0.00000T_Sep17-2014__14-58-58_001_091714.bin", "last mod"=timestamp(3493825138 s since 1904-01-01), "file name str"="D:\\Data\\Ultrasound\\LSCO\\LSCO22__130814c\\5_Cooling_2nd_try\\September_2014\\091714\\39.90500K_500_2500_2.10000V_0.00000T_Sep17-2014__14-58-58_001_091714.bin", "mod time(min)"=58230418.96666667, "file format"=enum."binary", "power(V)"=2.1, "Magn Field(T) "=0.0}, {"temperature"=39.827, "temperature str"="39.82700", "file path"=path "D:/Data/Ultrasound/LSCO/LSCO22__130814c/5_Cooling_2nd_try/September_2014/091714/39.82700K_500_2500_2.10000V_0.00000T_Sep17-2014__15-00-17_001_091714.bin", "last mod"=timestamp(3493825217 s since 1904-01-01), "file name str"="D:\\Data\\Ultrasound\\LSCO\\LSCO22__130814c\\5_Cooling_2nd_try\\September_2014\\091714\\39.82700K_500_2500_2.10000V_0.00000T_Sep17-2014__15-00-17_001_091714.bin", "mod time(min)"=58230420.28333333, "file format"=enum."binary", "power(V)"=2.1, "Magn Field(T) "=0.0}, {"temperature"=39.744, "temperature str"="39.74400", "file path"=path "D:/Data/Ultrasound/LSCO/LSCO22__130814c/5_Cooling_2nd_try/September_2014/091714/39.74400K_500_2500_2.10000V_0.00000T_Sep17-2014__15-01-36_001_091714.bin", "last mod"=timestamp(3493825296 s since 1904-01-01), "file name str"="D:\\Data\\Ultrasound\\LSCO\\LSCO22__130814c\\5_Cooling_2nd_try\\September_2014\\091714\\39.74400K_500_2500_2.10000V_0.00000T_Sep17-2014__15-01-36_001_091714.bin", "mod time(min)"=58230421.6, "file format"=enum."binary", "power(V)"=2.1, "Magn Field(T) "=0.0}, {"temperature"=39.665, "temperature str"="39.66500", "file path"=path "D:/Data/Ultrasound/LSCO/LSCO22__130814c/5_Co
